vi "messaging.vi"(8 "error in (no error)":errorcluster, 11 "Message_Control":T2) -> (0 "error out":errorcluster, 3 "REfs Out":T1)   [LabVIEW 2013]
doc: "Message FGV. Creates references for queues, based on thier Data Types. Has case to send init to all queues. Has case to get queue references, Has case to close queue refs.\n\nDeveloper must build cluster to hold queues, for the queue data types, use the module dat types for the queues and add the command enum for the module,"
uses:
  Error Handler/Error_Control.ctl
  Display Console/Display_Data.ctl
  Sensor Interface/Sensor_Station.ctl
  User Console/Requests.ctl
  Msg_Control.ctl
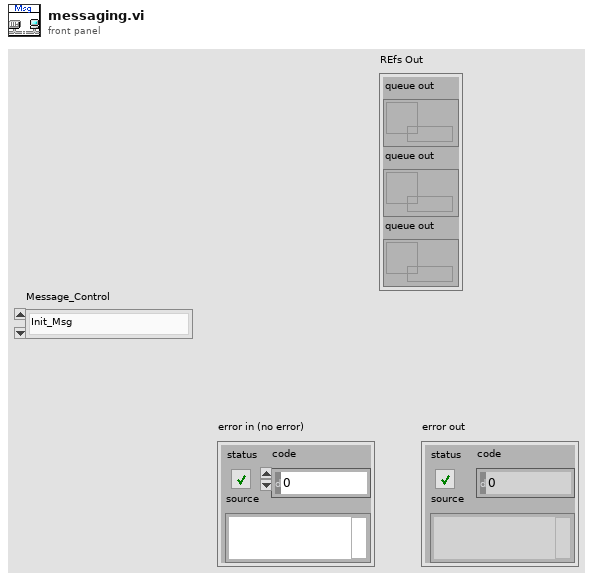
[diagram p1: front panel]
types:
  T1 = cluster{"queue out":refnum<queue>, "queue out":refnum<queue>, "queue out":refnum<queue>}
  T2 = typedef "Msg_Control.ctl" = enum16{"Init_Msg", "Sent_Inits", "Get_Ref", "Close_Ref"}
  T3 = typedef "Error_Control.ctl" = enum16{"Init", "Console_err", "Process_err", "Sensor_err"}
  T4 = typedef "Requests.ctl" = cluster{"1 u":bool, "3 u":bool, "2 u":bool, "2 d":bool, "4 d":bool, "3 d":bool, "1":bool, "2":bool, "3":bool, "4":bool}
  T5 = typedef "Sensor_Station.ctl" = u8
  T6 = typedef "Display_Data.ctl" = cluster{"Timing":dbl, "Current Floor":u8, "Up":bool, "Down":bool, "Door Open":bool, "Emergency":bool}
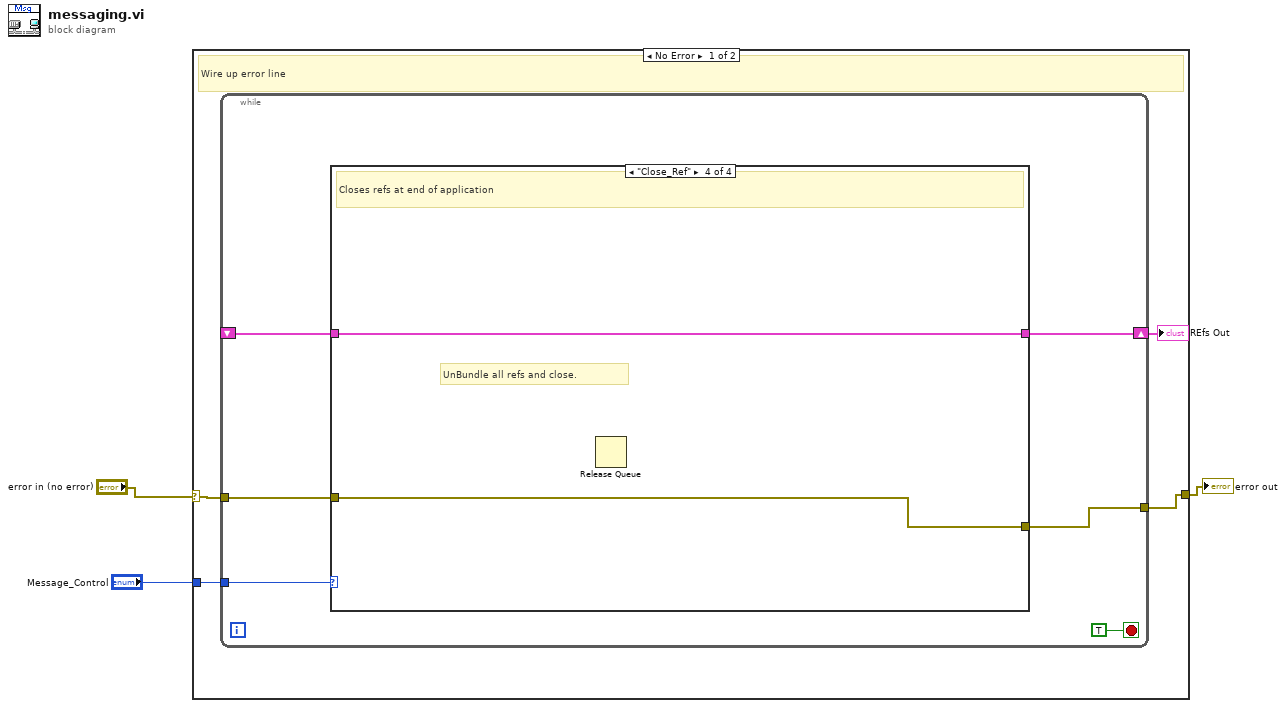
[diagram p0: block diagram]
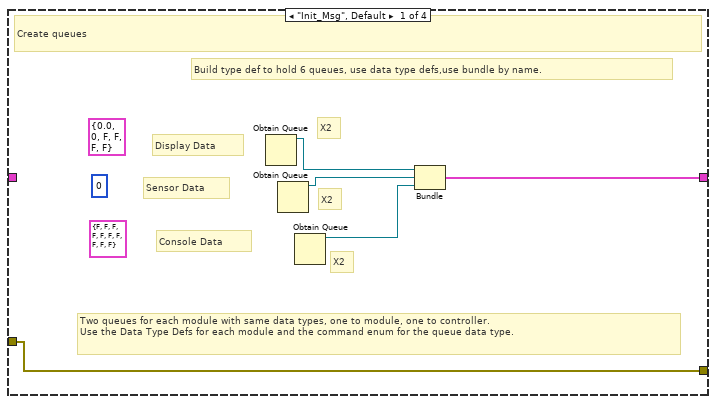
[diagram p2: hidden frame]
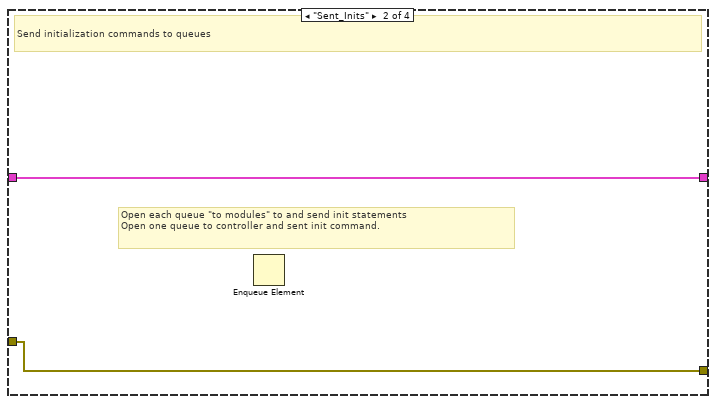
[diagram p3: hidden frame]
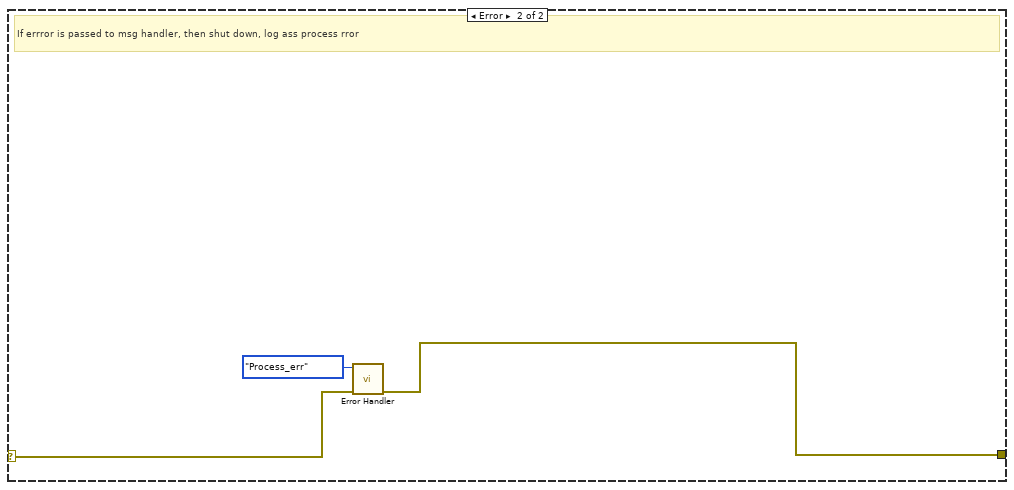
[diagram p5: hidden frame]
diagram:
  n1 = case shown="No Error" "error in (no error)" {
    selector: "error in (no error)" -> [w4 w27]
    tunnel: "Message_Control" -> [w7 _]
    tunnel: [w5 w26] -> w1
    frame No Error {
      # "Wire up error line"
      n2 = while {
        tunnel: w7 -> [w13]
        shift-right: [w11] -> w6
        shift-left: _ -> [w10]
        tunnel: [w9] -> w5
        tunnel: w4 -> [w8]
        stop <- TRUE stop-if-true
        n3 = case shown="\"Close_Ref\"" w13 {
          tunnel: [w15 _ _ _] -> w11
          tunnel: w10 -> [_ w20 w22 w24]
          tunnel: [_ w20 w22 w24] -> _
          tunnel: [w14 w19 w21 w23] -> w9
          tunnel: w8 -> [w14 w19 w21 w23]
          frame "Init_Msg", Default {
            (unwired) T4 {"1 u"=FALSE, "3 u"=FALSE, "2 u"=FALSE, "2 d"=FALSE, "4 d"=FALSE, "3 d"=FALSE, "1"=FALSE, "2"=FALSE, "3"=FALSE, "4"=FALSE} ("Requests")
            (unwired) T5 0 ("Slide")
            (unwired) T6 {"Timing"=0.0, "Current Floor"=0, "Up"=FALSE, "Down"=FALSE, "Door Open"=FALSE, "Emergency"=FALSE} ("Display_Data")
            # "X2"
            # "X2"
            # "X2"
            # "Console Data"
            # "Display Data"
            # "Sensor Data"
            # "Build type def to hold 6 queues, use data type defs,use bundle by name."
            # "Two queues for each module with same data types, one to module, one to controller.\nUse the Data Type Defs for each module and the command enum for the queue data type."
            # "Create queues"
            n4 = Obtain Queue() -> (queue out=w18:refnum<queue>)  [unwired: 5 in, 2 out]
            n5 = Obtain Queue() -> (queue out=w17:refnum<queue>)  [unwired: 5 in, 2 out]
            n6 = Obtain Queue() -> (queue out=w16:refnum<queue>)  [unwired: 5 in, 2 out]
            n7 = Bundle("queue out"=w18, "queue out"=w17, "queue out"=w16) -> (w15:T1)  [unwired: 1 in]
          }
          frame "Sent_Inits" {
            # "Open each queue \"to modules\" to and send init statements\nOpen one queue to controller and sent init command."
            # "Send initialization commands to queues"
            n8 = Enqueue Element() -> ()  [unwired: 4 in, 3 out]
          }
          frame "Get_Ref" {
            # "Just sends out the cluster of refs"
            # "Passes refs out to caller"
          }
          frame "Close_Ref" {
            # "UnBundle all refs and close."
            # "Closes refs at end of application"
            n9 = Release Queue() -> ()  [unwired: 3 in, 3 out]
          }
        }
      }
      "REfs Out" <- w6
    }
    frame Error {
      # "If errror is passed to msg handler, then shut down, log ass process rror"
      n10 = call "Error Handler.vi"("error in (no error)"=w27, "Error_Control"=Error_Control."Process_err") -> ("error out"=w26:errorcluster)  [unwired: 9 in]
    }
  }
  "error out" <- w1
